vi "Set Markers.vi"(0 "VISA Resource Name":refnum<visa-resource-name>, 1 "File Name (WAVEFORM_SEQ)":string="WAVEFORM_SEQ", 2 "Mark Number (1)":u16=1, 3 "First Point (1)":i32=1, 4 "Last Point (1)":i32=1, 5 "error in (no error)":errorcluster {"code" format="%.0x"}, 6 "Skip Count (0)":i32) -> (14 "VISA Resource Name Out":refnum<visa-resource-name>, 19 "error out":errorcluster {"code" format="%.0x"})   [LabVIEW 2012, in "Agilent ESG Series.lvlib"]
doc: "This VI defines a marker over a range of points on a waveform segment.\n\nNotes:\n(1) This VI is valid only on instruments Agilent E44xB with the UND option or on instrument E4438C with option 001/601 or 002/602."
uses:
  <instrlib>/Agilent ESG Series/Agilent ESG Series.lvlib
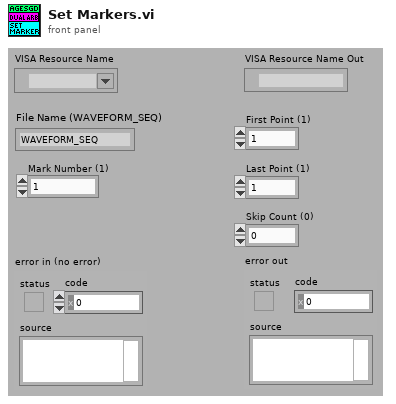
[diagram p1: front panel]
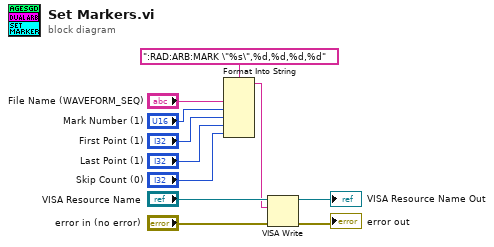
[diagram p0: block diagram]
diagram:
  n1 = Format Into String(format string=":RAD:ARB:MARK \"%s\",%d,%d,%d,%d", "File Name (WAVEFORM_SEQ)", "Mark Number (1)", "First Point (1)", "Last Point (1)", "Skip Count (0)") -> (resulting string=w1:string)  [unwired: 2 in, 1 out]
  n2 = VISA Write(VISA resource name="VISA Resource Name", write buffer=w1, error in (no error)="error in (no error)") -> (VISA resource name out=→"VISA Resource Name Out":refnum<visa-resource-name>, error out=→"error out":errorcluster)  [unwired: 1 out]
